vi "CrateMover 9001.vi"(3 "Crane Instructions":string[](array[string]), 5 "Cargo in":T1) -> (2 "Cargo out":T1)   [LabVIEW 2020, in "AoC 2022.lvlib"]
uses:
  AoC 2022.lvlib
  Cargo.ctl
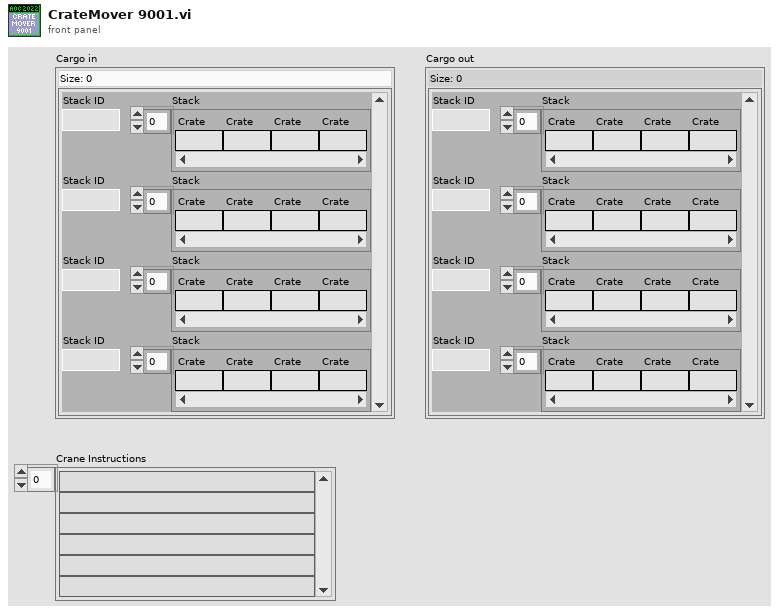
[diagram p1: front panel]
types:
  T1 = typedef "AoC 2022.lvlib/Cargo.ctl" = map{i32, string[]}
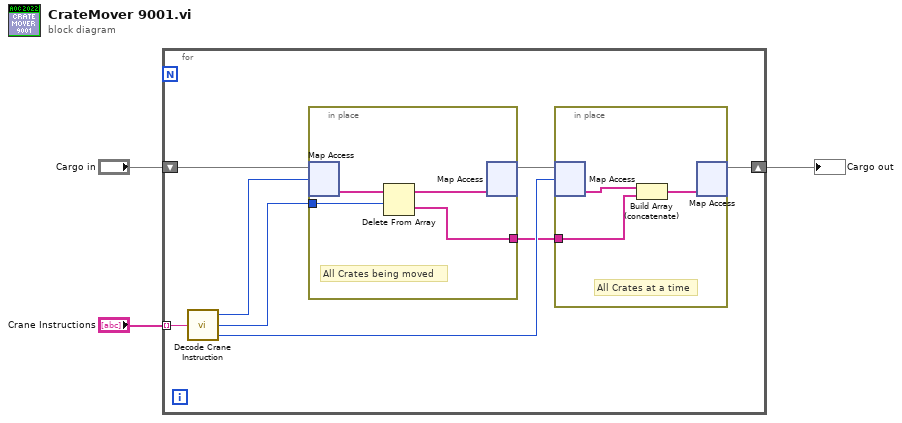
[diagram p0: block diagram]
diagram:
  n1 = for {
    tunnel: "Crane Instructions" -> [w11] mode=indexing
    shift-right: [w4] -> w3
    shift-left: "Cargo in" -> [w10]
    n2 = call "Decode Crane Instruction.vi"("Crane Instruction"=w11) -> ("From Stack"=w9:i32, "#Crates to be moved"=w8:i32, "To Stack"=w7:i32)
    n3 = in-place {
      in-place-border: w8 -> [w17]
      in-place-border: [w15] -> w5
      # "All Crates being moved"
      n4 = in-place-map #1(w10, w9) -> (w18:string[])  [unwired: 1 in, 1 out]
      n5 = Delete From Array(array=w18, length=w17) -> (deleted portion=w15:string[], array with subset deleted=w16:string[])  [unwired: 1 in]
      n6 = in-place-map #1(w16) -> (w6:T1)  [unwired: 1 in, 2 out]
    }
    n7 = in-place {
      in-place-border: w5 -> [w14]
      # "All Crates at a time"
      n8 = in-place-map #2(w6, w7) -> (w13:string[])  [unwired: 1 in, 1 out]
      n9 = Build Array (concatenate)(w13, w14) -> (w12:string[])
      n10 = in-place-map #2(w12) -> (w4:T1)  [unwired: 1 in, 2 out]
    }
  }
  "Cargo out" <- w3
